vi "Vision Processing.vi"(4 "error in (no error)":errorcluster, 7 "Image Size 2":T1=enum."320x240") -> ()   [LabVIEW 2017]
uses:
  <vilib>/Rock Robotics/WPI/Camera/WPI_CameraImageSize.ctl
  <vilib>/Rock Robotics/WPI/Camera/WPI_CameraWhite Balance Values.ctl
  <vilib>/Rock Robotics/WPI/Camera/WPI_CameraExposure Values.ctl
  <vilib>/Rock Robotics/WPI/Camera/WPI_CameraFrameRate.ctl
  Robot Global Data.vi
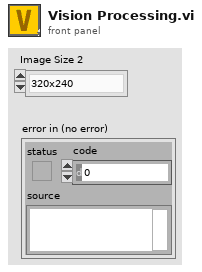
[diagram p1: front panel]
types:
  T1 = typedef "WPI_CameraImageSize.ctl" = enum16{"640x480", "320x240", "160x120", "Custom"}
  T2 = typedef "WPI_CameraFrameRate.ctl" = u32
  T3 = typedef "WPI_CameraExposure Values.ctl" = enum16{"Auto", "Flicker-free 50 Hz", "Flicker-free 60 Hz", "Hold current", "Custom"}
  T4 = typedef "WPI_CameraWhite Balance Values.ctl" = enum16{"Auto", "Fixed indoor", "Fixed outdoor 1", "Fixed outdoor 2", "Fixed fluorescent 1", "Fixed fluorescent 2", "Hold current", "Custom"}
  T5 = typedef "Image Type" = u32
  T6 = typedef "WPI_CameraDevRef.ctl" = cluster{"Camera Address":string, "CameraStatus":errorcluster}
  T7 = typedef "IMAQ Image.ctl" = refnum<image>
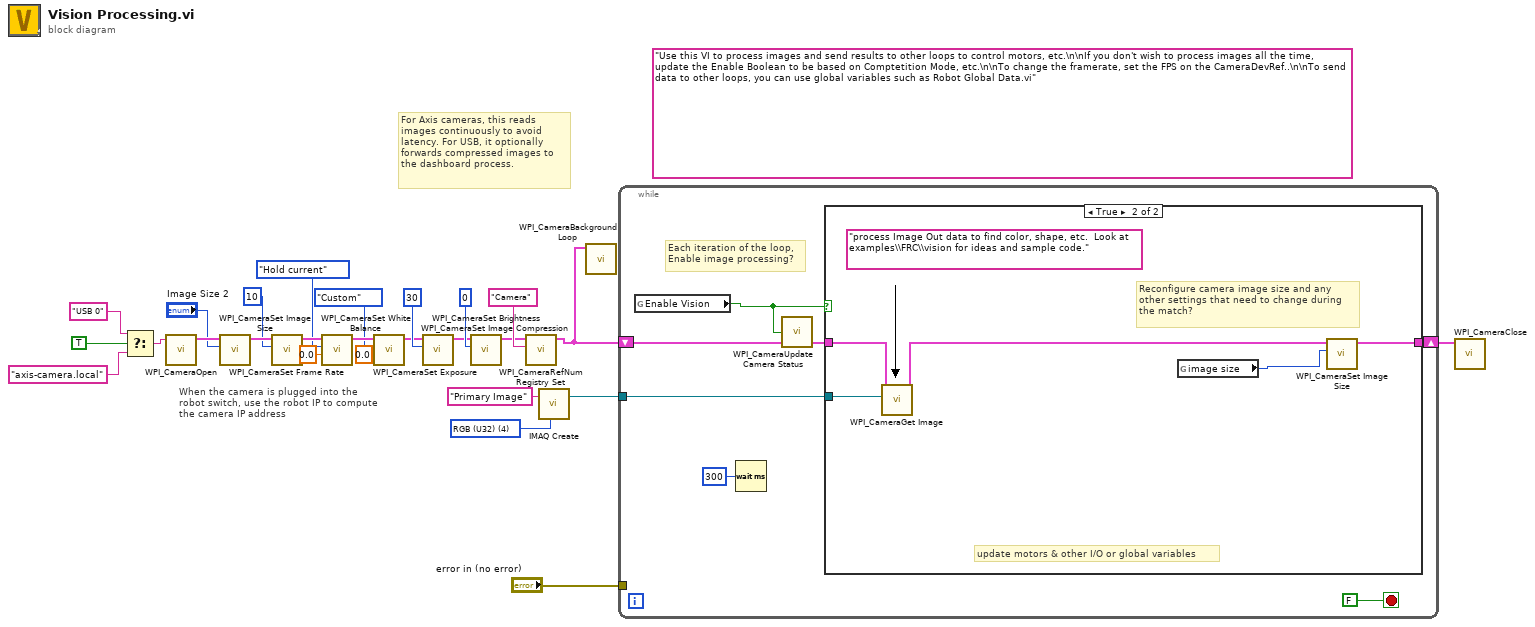
[diagram p0: block diagram]
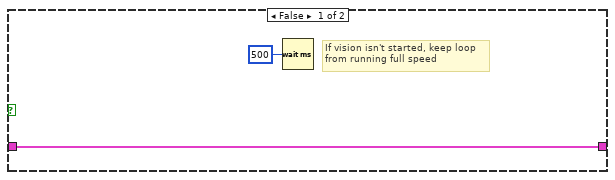
[diagram p2: hidden frame]
diagram:
  (unwired) "Use this VI to process images and send results to other loops to control motors, etc.\n\nIf you don't wish to process images all the time, update the Enable Boolean to be based on Comptetition Mode, etc.\n\nTo change the framerate, set the FPS on the CameraDevRef..\n\nTo send data to other loops, you can use global variables such as Robot Global Data.vi"
  w26 = T5 4 items=["Grayscale (U8)", "Grayscale (I16)", "Grayscale (SGL)", "Complex (CSG)", "RGB (U32)", "HSL (U32)", "RGB (U64)"] ("Image Type")
  # "When the camera is plugged into the\nrobot switch, use the robot IP to compute\nthe camera IP address"
  # "For Axis cameras, this reads\nimages continuously to avoid\nlatency. For USB, it optionally\nforwards compressed images to\nthe dashboard process."
  n1 = Select(t="USB 0" ("format string"), s=TRUE ("dot notation? (F)"), f="axis-camera.local" ("format string")) -> (s? t:f=w2:string)
  n2 = call <vilib>:"WPI_CameraOpen.vi"("Camera Address"=w2) -> ("CameraDevRef"=w10:T6)  [unwired: 1 in, 9 out]
  n3 = call <vilib>:"WPI_CameraSet Image Size.vi"("Image Size"="Image Size 2", "CameraDevRef"=w10) -> ("CameraDevRef Out"=w11:T6)  [unwired: 2 in, 7 out]
  n4 = call <vilib>:"WPI_CameraSet Frame Rate.vi"("Frame Rate (fps)"=T2 10, "CameraDevRef"=w11) -> ("CameraDevRef Out"=w13:T6)  [unwired: 1 in, 8 out]
  n5 = call <vilib>:"WPI_CameraSet White Balance.vi"("Color Temp (K)"=0.0, "White Balance"=WPI_CameraWhite_Balance_Values."Hold current", "CameraDevRef"=w13) -> ("CameraDevRef Out"=w12:T6)  [unwired: 1 in, 7 out]
  n6 = call <vilib>:"WPI_CameraSet Exposure.vi"("Exposure (%)"=0.0, "Exposure"=WPI_CameraExposure_Values."Custom", "CameraDevRef"=w12) -> ("CameraDevRef Out"=w15:T6)  [unwired: 1 in, 7 out]
  n7 = call <vilib>:"WPI_CameraSet Image Compression.vi"("Compression"=30, "CameraDevRef"=w15) -> ("CameraDevRef Out"=w14:T6)  [unwired: 1 in, 8 out]
  n8 = call <vilib>:"WPI_CameraSet Brightness.vi"("Brightness"=0, "CameraDevRef"=w14) -> ("CameraDevRef Out"=w9:T6)  [unwired: 2 in, 7 out]
  n9 = call <vilib>:"WPI_CameraRefNum Registry Set.vi"("refnum name"="Camera", "CameraDevRef"=w9) -> ("CameraDevRef"=w1:T6)  [unwired: 2 in, 7 out]
  n10 = call "IMAQ Create"("Image Name"="Primary Image", "Image Type"=w26) -> ("New Image"=w24:T7)  [unwired: 2 in, 2 out]
  n11 = call <vilib>:"WPI_CameraBackground Loop.vi"("CameraDevRef"=w1) -> ()  [unwired: 11 in]
  n12 = while {
    shift-right: [w32] -> w23
    shift-left: w1 -> [w30]
    tunnel: w24 -> [w31]
    tunnel: "error in (no error)" -> [_]
    stop <- FALSE stop-if-true
    # "Each iteration of the loop,\nEnable image processing?"
    n13 = global read "Robot Global Data.vi" "Enable Vision"() -> (w28:bool)
    n14 = Wait (ms)(milliseconds to wait=u32 300) -> ()  [unwired: 1 out]
    n15 = call <vilib>:"WPI_CameraUpdate Camera Status.vi"("CameraDevRef In"=w30, "Enable Vision"=w28) -> ("CameraDevRef Out"=w29:T6)  [unwired: 3 in]
    n16 = case shown="True" w28 {
      tunnel: w31 -> [_ w39]
      tunnel: [w35 w40] -> w32
      tunnel: w29 -> [w35 w38]
      frame False {
        # "If vision isn't started, keep loop\nfrom running full speed"
        n17 = Wait (ms)(milliseconds to wait=u32 500) -> ()  [unwired: 1 out]
      }
      frame True {
        (unwired) "process Image Out data to find color, shape, etc.  Look at examples\\FRC\\vision for ideas and sample code."
        # "update motors & other I/O or global variables"
        # "Reconfigure camera image size and any\nother settings that need to change during\nthe match?"
        n18 = call <vilib>:"WPI_CameraGet Image.vi"("Image"=w39, "CameraDevRef"=w38) -> ("CameraDevRef Out"=w37:T6)  [unwired: 1 in, 8 out]
        n19 = global read "Robot Global Data.vi" "image size"() -> (w36:T1)
        n20 = call <vilib>:"WPI_CameraSet Image Size.vi"("Image Size"=w36, "CameraDevRef"=w37) -> ("CameraDevRef Out"=w40:T6)  [unwired: 2 in, 7 out]
      }
    }
  }
  n21 = call <vilib>:"WPI_CameraClose.vi"("CameraDevRef"=w23) -> ()  [unwired: 1 in, 10 out]
